vi "curvature-cator - i.vi"(0 "omega array in":dbl[](array[numeric]), 1 "size":i32=1, 2 "number of grid points":i32=300, 3 "decimation threshold":i32=3, 5 "z array in":cdb[](array[numeric]), 9 "wavepacket in":T3={"R"=0.5, "wave number"=22.0, "delta k"=7.0, "radii vector"=[], "radial section"=[], "wave vector"=22.0, "wavepacket is"=TRUE} {"delta k" format="%#_3f"; "wave number" format="%#_3f"; "R" format="%#_3f"}, 11 "scale factor":dbl=3.0, 12 "first time":bool, 13 "main VI path":path) -> (4 "spot center":cdb, 6 "spot size":dbl, 10 "4 corners rescaled out":T2={"z (-pi/2)"=-1.0311345636926572+0.5736824521422934i, "z(inf)"=-0.5200164984937075+1.0975277942502903i, "z (pi/2)"=-1.0311345636926572+0.5736824521422934i, "z center"=-0.5136528600391839+0.580046090596817i, "z(0)"=-0.5200164984937075+1.0975277942502903i, "radius"=-1.0311345636926572}, 15 "lorentzian out":T1={"Amplitude"=-1.0311345636926572, "omega(0)"=-1.0311345636926572, "Gamma"=-1.0311345636926572, "phase"=-1.0311345636926572, "Q"=-1.0311345636926572, "Norm  Ampl"=-1.0311345636926572, "z (inf)"=-1.0311345636926572+0.0i, "4corners"={"z (-pi/2)"=-1.0311345636926572+0.5736824521422934i, "z(inf)"=-0.5200164984937075+1.0975277942502903i, "z (pi/2)"=-1.0311345636926572+0.5736824521422934i, "z center"=-0.5136528600391839+0.580046090596817i, "z(0)"=-0.5200164984937075+1.0975277942502903i, "radius"=-1.0311345636926572}} {"z (inf)" format="%#9_9f"; "Q" format="%#9_9f"; "phase" format="%#9_9f"; "Gamma" format="%#9_9f"; "omega(0)" format="%#9_9f"})   [LabVIEW 2010]
uses:
  wavepacket.ctl
  circle corners.ctl
  lorentzian.ctl
  complex region.ctl
  <vilib>/Analysis/baseanly.llb/Median.vi
  <vilib>/Analysis/baseanly.llb/Mean.vi
  <vilib>/Analysis/2dsp.llb/Unwrap Phase.vi
  <vilib>/gmath/NumericalOptimization/Nonlinear Curve Fit.vi
  <vilib>/gmath/NumericalOptimization/Nonlinear Curve Fit LM.vi
  <vilib>/Utility/error.llb/Clear Errors.vi
panel:
  out "mean":cdb
  in  "number":cdb
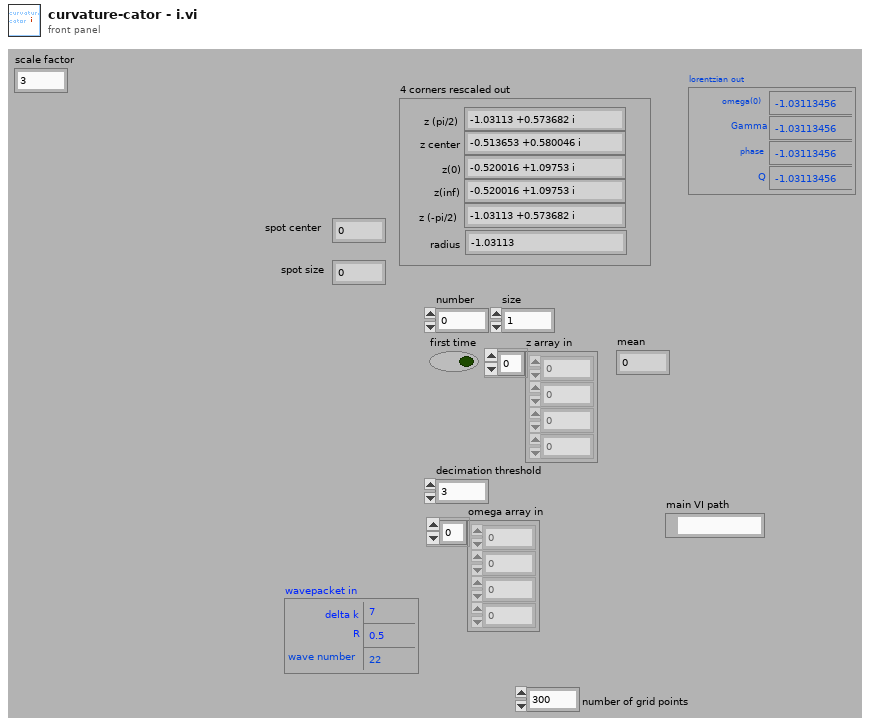
[diagram p1: front panel]
types:
  T1 = typedef "lorentzian.ctl" = cluster{"Amplitude":dbl, "omega(0)":dbl, "Gamma":dbl, "phase":dbl, "Q":dbl, "Norm  Ampl":dbl, "z (inf)":cdb, "4corners":T2}
  T2 = typedef "circle corners.ctl" = cluster{"z (-pi/2)":cdb, "z(inf)":cdb, "z (pi/2)":cdb, "z center":cdb, "z(0)":cdb, "radius":dbl}
  T3 = typedef "wavepacket.ctl" = cluster{"R":dbl, "wave number":dbl, "delta k":dbl, "radii vector":dbl[], "radial section":cdb[], "wave vector":dbl, "wavepacket is":bool}
  T4 = typedef "complex region.ctl" = cluster{"max re":dbl, "min re":dbl, "max im":dbl, "min im":dbl, "delta re":dbl, "delta im":dbl, "center re":dbl, "delta  z":cdb, "center im":dbl, "center z":cdb, "d im":dbl, "d re":dbl, "d z":cdb}
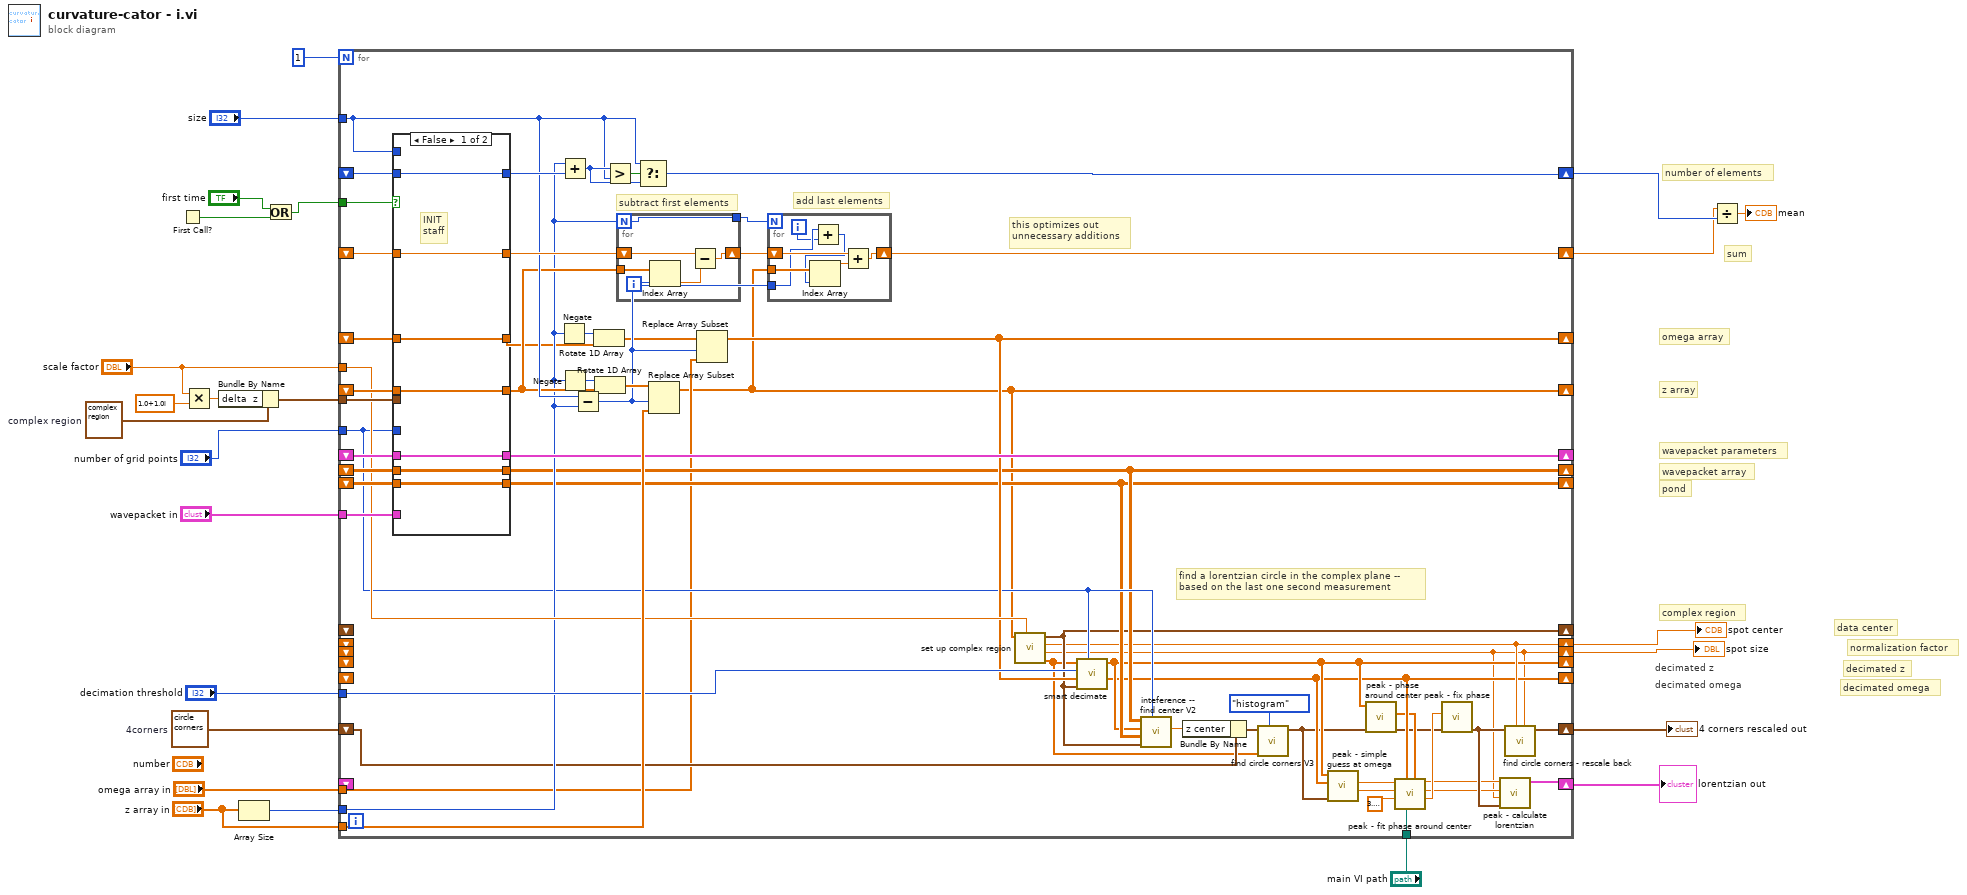
[diagram p0: block diagram]
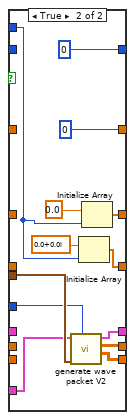
[diagram p2: hidden frame]
diagram:
  w16 = T4 {"max re"=1.5, "min re"=-1.5, "max im"=1.5, "min im"=-1.5, "delta re"=3.0, "delta im"=3.0, "center re"=0.0, "delta  z"=3.0+3.0i, "center im"=0.0, "center z"=0.0+0.0i, "d im"=0.0, "d re"=0.0, "d z"=0.0+0.0i}  # complex region
  w13 = T2 {"z (-pi/2)"=-1.0311345636926572+0.5736824521422934i, "z(inf)"=-0.5200164984937075+1.0975277942502903i, "z (pi/2)"=-1.0311345636926572+0.5736824521422934i, "z center"=-0.5136528600391839+0.580046090596817i, "z(0)"=-0.5200164984937075+1.0975277942502903i, "radius"=-1.0311345636926572}  # 4corners
  # "decimated omega"
  # "decimated z"
  # "decimated omega"
  # "decimated z"
  # "omega array"
  # "normalization factor"
  # "data center"
  # "pond"
  # "wavepacket array"
  # "wavepacket parameters"
  # "complex region"
  # "z array"
  # "sum"
  # "number of elements"
  n1 = First Call?() -> (First Call?: T/F=w7:bool)
  n2 = Multiply(x="scale factor", y=cdb 1.0+1.0i) -> (x*y=w3:cdb)
  n3 = Bundle By Name(cluster=w16, "delta  z"=w3) -> (w15:T4)
  n4 = Array Size(array="z array in") -> (size(s)=w21:i32)
  n5 = Or(x="first time", y=w7) -> (x .or. y?=w6:bool)
  n6 = for {
    N: 1 -> [_]
    tunnel: w6 -> [w76]
    shift-right: [w70] -> w19
    shift-left: _ -> [w81]
    shift-right: [w82] -> w23
    shift-left: _ -> [w84]
    tunnel: "size" -> [w73]
    shift-right: [w40] -> _
    shift-left: _ -> [w78]
    tunnel: w21 -> [w57]
    tunnel: "z array in" -> [w72]
    tunnel: "number of grid points" -> [w53]
    tunnel: "wavepacket in" -> [w69]
    shift-right: [w52] -> _
    shift-left: _ -> [w65]
    shift-right: [w51] -> _
    shift-left: _ -> [w64]
    shift-right: [w68] -> _
    shift-left: _ -> [w66]
    tunnel: w15 -> [w67]
    shift-right: [w50] -> _
    shift-left: _ -> [_]
    tunnel: "scale factor" -> [w62]
    shift-right: [w41] -> w11
    shift-left: _ -> [_]
    shift-right: [w26] -> w10
    shift-left: _ -> [_]
    tunnel: "decimation threshold" -> [w61]
    shift-right: [w54] -> _
    shift-left: _ -> [w60]
    shift-right: [w35] -> _
    shift-left: _ -> [_]
    shift-right: [w34] -> _
    shift-left: _ -> [_]
    shift-right: [w42] -> w9
    shift-left: w13 -> [w48]
    tunnel: "omega array in" -> [w45]
    tunnel: "main VI path" -> [w31]
    shift-right: [w30] -> w1
    shift-left: _ -> [_]
    # "find a lorentzian circle in the complex plane -- \nbased on the last one second measurement"
    # "add last elements"
    # "subtract first elements"
    # "this optimizes out \nunnecessary additions"
    n7 = case shown="False" w76 {
      tunnel: w84 -> [w104 _]
      tunnel: w81 -> [w102 _]
      tunnel: [w102 0] -> w74
      tunnel: [w104 0] -> w80
      tunnel: w78 -> [w103 _]
      tunnel: [w103 w116] -> w63
      tunnel: w73 -> [_ w112]
      tunnel: w53 -> [_ w109]
      tunnel: w69 -> [_ w108]
      tunnel: [w99 w106] -> w52
      tunnel: [w98 w105] -> w51
      tunnel: [w100 w107] -> w68
      tunnel: w67 -> [_ w110]
      tunnel: w66 -> [w100 _]
      tunnel: w65 -> [w99 _]
      tunnel: w64 -> [w98 _]
      tunnel: [w101 w111] -> w56
      tunnel: w60 -> [w101 _]
      frame False {
        # "INIT\nstaff"
      }
      frame True {
        n8 = call "generate wave packet V2.vi"("number of grid points"=w109, "complex region"=w110, "wavepacket in"=w108) -> ("pond array out"=w105:cdb[][], "wavepacket array out"=w106:cdb[][], "wavepacket out"=w107:T3)  [unwired: 6 in]
        n9 = Initialize Array(cdb 0.0+0.0i, w112) -> (w116:cdb[])
        n10 = Initialize Array(0.0, w112) -> (w111:dbl[])
      }
    }
    n11 = Negate(x=w57) -> (-x=w58:i32)
    n12 = Add(x=w57, y=w80) -> (x+y=w79:i32)
    n13 = Negate(x=w57) -> (-x=w75:i32)
    n14 = Subtract(x=w73, y=w57) -> (x-y=w59:i32)
    n15 = Rotate 1D Array(1:w56, 2:w58) -> (0:w55:dbl[])
    n16 = Rotate 1D Array(1:w63, 2:w75) -> (0:w77:cdb[])
    n17 = Greater?(x=w79, y=w73) -> (0:w83:bool)
    n18 = for {
      N: w57 -> [w92]
      tunnel: w63 -> [w96]
      shift-right: [w93] -> w71
      shift-left: w74 -> [w97]
      tunnel: [w92] -> w43
      i -> [w95]
      n19 = Index Array(array=w96, index=w95) -> (element=w94:cdb)
      n20 = Subtract(x=w97, y=w94) -> (x-y=w93:cdb)
    }
    n21 = Select(t=w73, s=w83, f=w79) -> (s? t:f=w82:i32)
    n22 = Replace Array Subset(array=w77, new element=w72, index=w59) -> (w40:cdb[])
    n23 = Replace Array Subset(array=w55, new element=w45, index=w59) -> (w54:dbl[])
    n24 = for {
      N: w43 -> [_]
      shift-right: [w89] -> w70
      shift-left: w71 -> [w91]
      tunnel: w40 -> [w88]
      tunnel: w59 -> [w86]
      i -> [w85]
      n25 = Add(x=w86, y=w85) -> (x+y=w87:i32)
      n26 = Index Array(array=w88, index=w87) -> (element=w90:cdb)
      n27 = Add(x=w91, y=w90) -> (x+y=w89:cdb)
    }
    n28 = call "set up complex region.vi"("scale factor"=w62, "z in window"=w40) -> ("z  normalized"=w44:cdb[], "normalization factor"=w26:dbl, "data center"=w41:cdb, "complex region"=w50:T4)  [unwired: 6 in]
    n29 = call "smart decimate .vi"("number of 2D grid points"=w53, "complex region"=w50, "omega in"=w54, "decimation threshold"=w61, "z in"=w44) -> ("decimated omega"=w34:dbl[], "decimated z"=w35:cdb[])  [unwired: 5 in]
    n30 = call "inteference -- find center V2.vi"("number of points"=w53, "complex region"=w50, "pond"=w51, "point sources"=w35, "wave packet"=w52) -> ("z (center)"=w49:cdb)  [unwired: 6 in]
    n31 = Bundle By Name(cluster=w48, "z center"=w49) -> (w47:T2)
    n32 = call "find circle corners V3.vi"("method"=enum16{"median", "method 2", "histogram"}."histogram", "z"=w44, "circle corners in"=w47) -> ("circle corners out"=w32:T2)  [unwired: 8 in]
    n33 = call "peak - simple guess at omega.vi"("4corners"=w32, "decimated omega"=w34, "z"=w35) -> ("Gamma"=w38:dbl, "guess at omega"=w39:dbl)  [unwired: 7 in]
    n34 = call "peak - phase around center.vi"("4corners"=w32, "decimated z"=w35) -> ("Unwrapped Phase"=w33:dbl[])  [unwired: 9 in]
    n35 = call "peak - fit phase around center.vi"("Unwrapped Phase"=w33, "main VI  path"=w31, "decimated omega"=w34, "guess at theta"=3.141592653589793, "guess at gamma"=w38, "guess at omega"=w39) -> ("fit for theta"=w36:dbl, "fit for gamma"=w27:dbl, "fit for omega"=w28:dbl)  [unwired: 3 in]
    n36 = call "peak - fix phase.vi"("4corners"=w32, "correct phase"=w36) -> ("4corners out"=w29:T2)  [unwired: 9 in]
    n37 = call "peak - calculate lorentzian.vi"("4corners"=w29, "normalization factor"=w26, "gamma"=w27, "omega"=w28) -> ("lorentzian out"=w30:T1)  [unwired: 7 in]
    n38 = call "find circle corners - rescale back.vi"("spot size"=w26, "spot center"=w41, "4 corners in"=w29) -> ("4 corners out"=w42:T2)  [unwired: 8 in]
  }
  "spot center" <- w11
  "spot size" <- w10
  "4 corners rescaled out" <- w9
  "lorentzian out" <- w1
  n39 = Divide(x=w19, y=w23) -> (x/y=→"mean":cdb)
